vi "test_request_builder_api.vi"() -> ()   [LabVIEW 2020, in "reqwest_tests.lvlib"]
uses:
  reqwest_tests.lvlib
  <vilib>/addons/_JKI Toolkits/Caraya/classes/Assert/Assert.lvclass
  <vilib>/addons/_JKI Toolkits/Caraya/classes/Test/Test.lvclass
  ClientBuilder/ClientBuilder.lvclass
  Client/Client.lvclass
  Types/http_method_enum.ctl
  reqwest.lvlib
  RequestBuilder/RequestBuilder.lvclass
  Headers/Headers.lvclass
  Request/Request.lvclass
panel:
  out "string_value":string
  out "is_complete":bool
  in  "error in (no error)":errorcluster
  out "error out":errorcluster
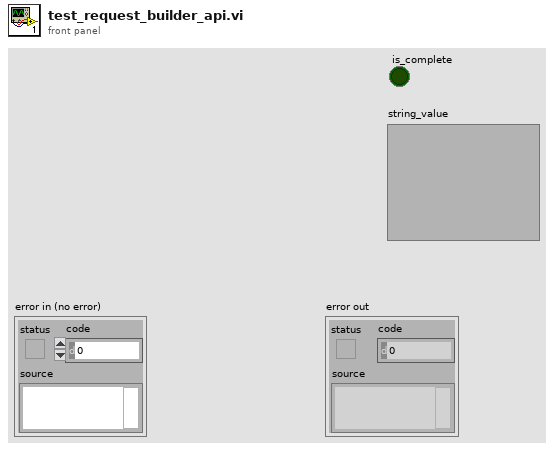
[diagram p1: front panel]
types:
  T1 = typedef "reqwest.lvlib/http_method_enum.ctl" = enum8{"<select>", "GET", "POST", "PUT", "DELETE", "HEAD", "OPTIONS", "CONNECT", "PATCH", "TRACE"}
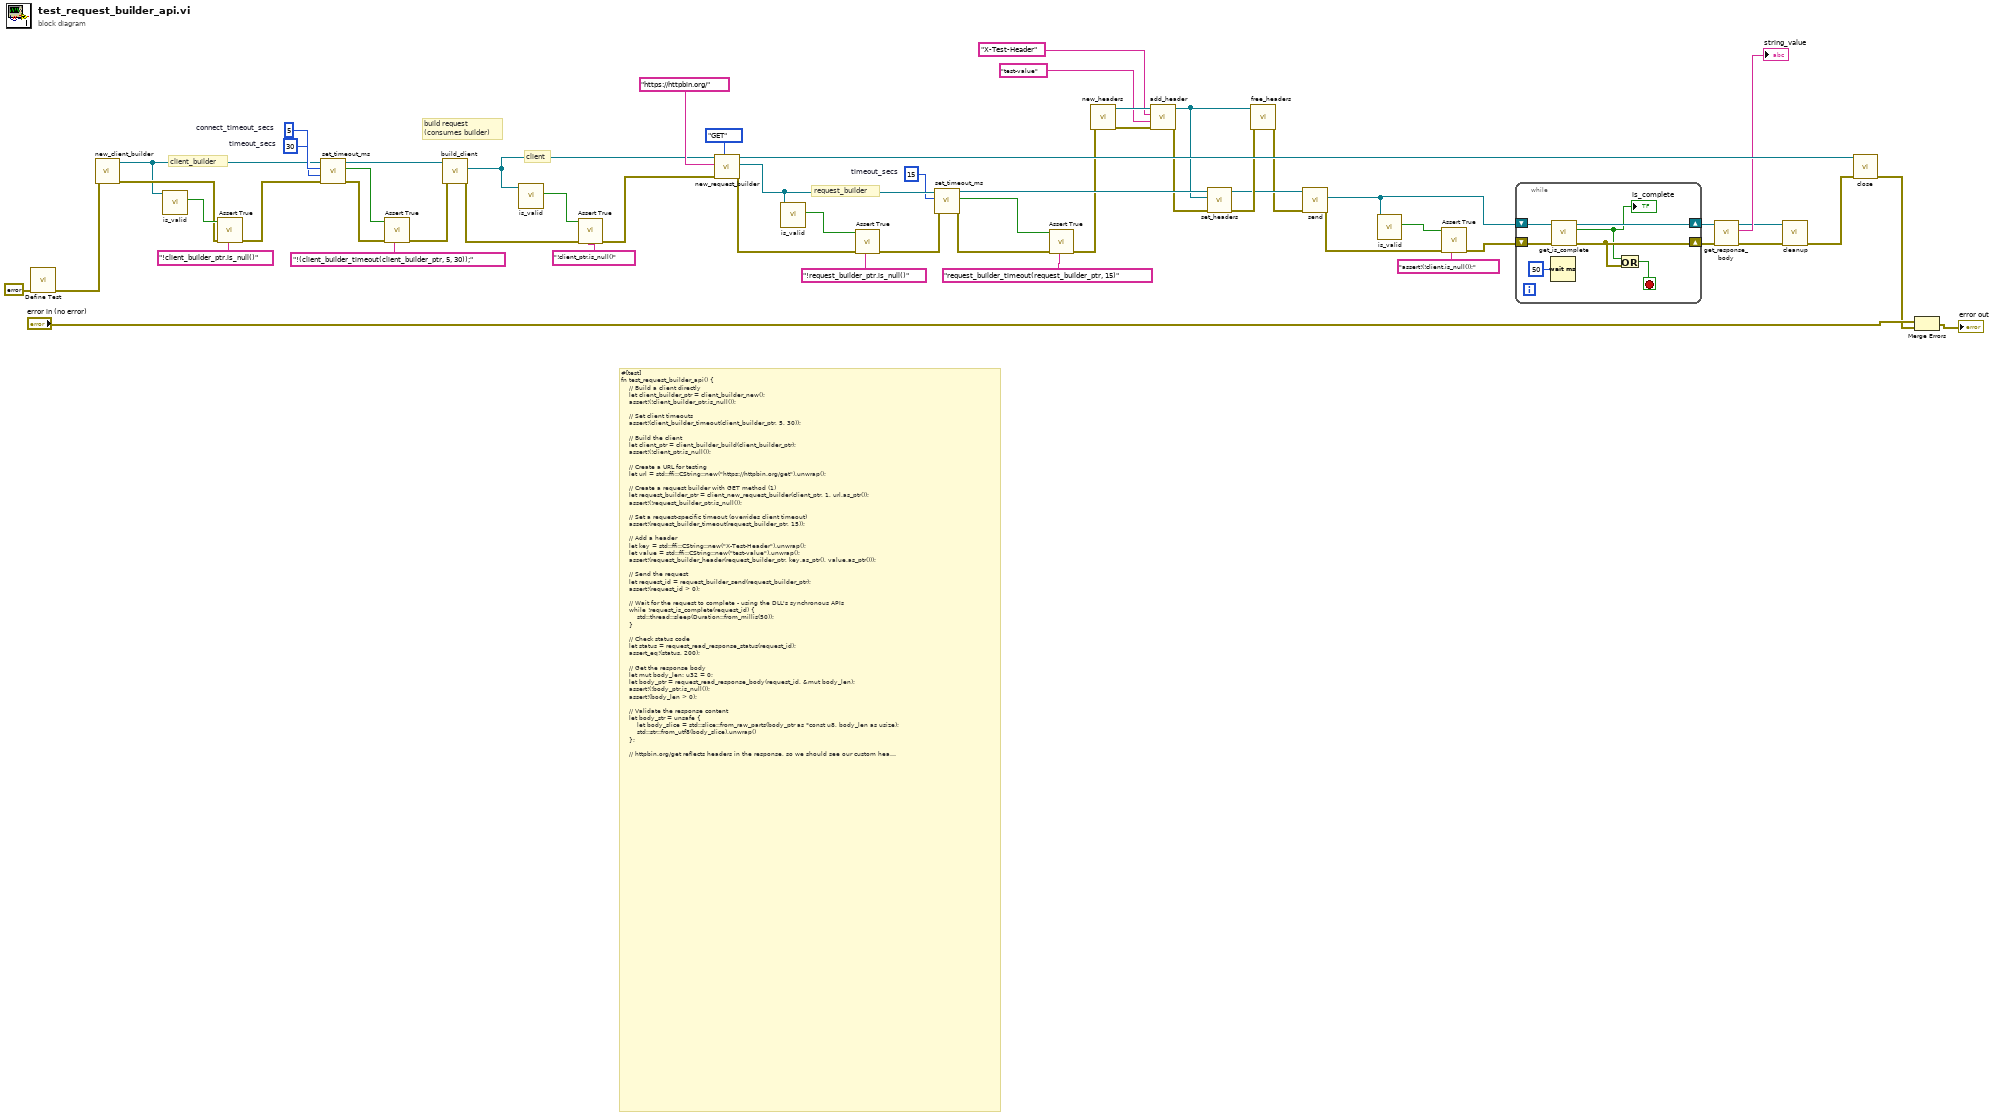
[diagram p0: block diagram]
diagram:
  w30 = u64 15  # timeout_secs
  w45 = u64 30  # timeout_secs
  w46 = u64 5  # connect_timeout_secs
  # "request_builder"
  # "client"
  # "client_builder"
  # "build request\n(consumes builder)"
  # "#[test]\nfn test_request_builder_api() {\n    // Build a client directly \n    let client_builder_ptr = client_builder_new();\n    assert!(!client_builder_ptr.is_null());\n    \n    // Set client timeouts\n    assert!(client_builder_timeout(client_builder_ptr, 5, 30));\n    \n    // Build the client\n    let client_ptr = client_builder_build(client_builder_ptr);\n    assert!(!client_ptr.is_null());\n\n    // Create a URL for testing\n    let url = std::ffi::CString::new(\"https://httpbin.org/get\").unwrap();\n    \n    // Create a request builder with GET method (1)\n    let request_builder_ptr = client_new_request_builder(client_ptr, 1, url.as_ptr());\n    assert!(!request_builder_ptr.is_null());\n    \n    // Set a request-specific timeout (overrides client timeout)\n    assert!(request_builder_timeout(request_builder_ptr, 15));\n    \n    // Add a header\n    let key = std::ffi::CString::new(\"X-Test-Header\").unwrap();\n    let value = std::ffi::CString::new(\"test-value\").unwrap();\n    assert!(request_builder_header(request_builder_ptr, key.as_ptr(), value.as_ptr()));\n    \n    // Send the request\n    let request_id = request_builder_send(request_builder_ptr);\n    assert!(request_id > 0);\n    \n    // Wait for the request to complete - using the DLL's synchronous APIs\n    while !request_is_complete(request_id) {\n        std::thread::sleep(Duration::from_millis(50));\n    }\n    \n    // Check status code\n    let status = request_read_response_status(request_id);\n    assert_eq!(status, 200);\n    \n    // Get the response body\n    let mut body_len: u32 = 0;\n    let body_ptr = request_read_response_body(request_id, &mut body_len);\n    assert!(!body_ptr.is_null());\n    assert!(body_len > 0);\n    \n    // Validate the response content\n    let body_str = unsafe {\n        let body_slice = std::slice::from_raw_parts(body_ptr as *const u8, body_len as usize);\n        std::str::from_utf8(body_slice).unwrap()\n    };\n    \n    // httpbin.org/get reflects headers in the response, so we should see our custom header\n    assert!(body_str.contains(\"X-Test-Header\"));\n    assert!(body_str.contains(\"test-value\"));\n    \n    // Cleanup\n    free_memory(body_ptr);\n    request_cleanup(request_id);\n    client_close(client_ptr);\n}"
  n1 = call <vilib>:"Define Test.vi"("error in (no error)"=errorcluster {"status"=FALSE, "code"=0, "source"=""}) -> ("error out"=w48:errorcluster)  [unwired: 9 in, 1 out]
  n2 = call "new_client_builder.vi"("error in (no error)"=w48) -> ("error out"=w47:errorcluster, "Client out"=w41:refnum<class "ClientBuilder.lvclass">)  [unwired: 9 in]
  n3 = call "is_valid.vi"("Client in"=w41) -> ("valid-ref?"=w53:bool)  [unwired: 10 in]
  n4 = call <vilib>:"Assert True.vi"("Label"="!client_builder_ptr.is_null()", "error in (no error)"=w47, "True?"=w53) -> ("error out"=w40:errorcluster)  [unwired: 7 in, 1 out]
  n5 = call "set_timeout_ms.vi"("error in (no error)"=w40, "timeout_secs"=w45, 10:w46, "ClientBuilder in"=w41) -> ("error out"=w42:errorcluster, "success"=w43:bool, "ClientBuilder out"=w38:refnum<class "ClientBuilder.lvclass">)  [unwired: 5 in]
  n6 = call <vilib>:"Assert True.vi"("Label"="!(client_builder_timeout(client_builder_ptr, 5, 30));", "error in (no error)"=w42, "True?"=w43) -> ("error out"=w26:errorcluster)  [unwired: 7 in, 1 out]
  n7 = call "build_client.vi"("error in (no error)"=w26, "ClientBuilder in"=w38) -> ("error out"=w25:errorcluster, "Client out"=w34:refnum<class "Client.lvclass">)  [unwired: 8 in]
  n8 = call "is_valid.vi"("Client in"=w34) -> ("valid-ref?"=w51:bool)  [unwired: 10 in]
  n9 = call <vilib>:"Assert True.vi"("Label"="!client_ptr.is_null()", "error in (no error)"=w25, "True?"=w51) -> ("error out"=w32:errorcluster)  [unwired: 7 in, 1 out]
  n10 = call "new_request_builder.vi"("HTTP Method"=http_method_enum."GET", "error in (no error)"=w32, "url"="https://httpbin.org/" ("Label"), "Client in"=w34) -> ("error out"=w24:errorcluster, "RequestBuilder out"=w31:refnum<class "RequestBuilder.lvclass">, "Client out"=w33:refnum<class "Client.lvclass">)  [unwired: 5 in]
  n11 = call "is_valid.vi"("obj in"=w31) -> ("valid-ref?"=w35:bool)  [unwired: 10 in]
  n12 = call <vilib>:"Assert True.vi"("Label"="!request_builder_ptr.is_null()", "error in (no error)"=w24, "True?"=w35) -> ("error out"=w23:errorcluster)  [unwired: 7 in, 1 out]
  n13 = call "set_timeout_ms.vi"("error in (no error)"=w23, "timeout_ms"=w30, "obj in"=w31) -> ("error out"=w27:errorcluster, "success"=w28:bool, "obj out"=w22:refnum<class "RequestBuilder.lvclass">)  [unwired: 6 in]
  n14 = call <vilib>:"Assert True.vi"("Label"="request_builder_timeout(request_builder_ptr, 15)", "error in (no error)"=w27, "True?"=w28) -> ("error out"=w15:errorcluster)  [unwired: 7 in, 1 out]
  n15 = call "new_headers.vi"("error in (no error)"=w15) -> ("error out"=w18:errorcluster, "Headers out"=w21:refnum<class "Headers.lvclass">)  [unwired: 9 in]
  n16 = call "add_header.vi"("error in (no error)"=w18, "value"="test-value" ("Label"), "key"="X-Test-Header" ("Label"), "Headers in"=w21) -> ("error out"=w16:errorcluster, "Headers out"=w17:refnum<class "Headers.lvclass">)  [unwired: 5 in, 1 out]
  n17 = call "set_headers.vi"("error in (no error)"=w16, "Headers"=w17, "obj in"=w22) -> ("error out"=w14:errorcluster, "obj out"=w13:refnum<class "RequestBuilder.lvclass">)  [unwired: 6 in, 1 out]
  n18 = call "free_headers.vi"("error in (no error)"=w14, "Headers in"=w17) -> ("error out"=w5:errorcluster)  [unwired: 9 in]
  n19 = call "send.vi"("error in (no error)"=w5, "obj in"=w13) -> ("error out"=w4:errorcluster, "request"=w6:refnum<class "Request.lvclass">)  [unwired: 8 in]
  n20 = call "is_valid.vi"("Request in"=w6) -> ("valid-ref?"=w11:bool)  [unwired: 10 in]
  n21 = call <vilib>:"Assert True.vi"("Label"="assert!(!client.is_null());", "error in (no error)"=w4, "True?"=w11) -> ("error out"=w10:errorcluster)  [unwired: 7 in, 1 out]
  n22 = while {
    shift-right: [w63] -> w7
    shift-left: w6 -> [w62]
    shift-right: [w59] -> w9
    shift-left: w10 -> [w60]
    stop <- w57 stop-if-true
    n23 = Wait (ms)(milliseconds to wait=u32 50) -> ()  [unwired: 1 out]
    n24 = call "get_is_complete.vi"("error in (no error)"=w60, "Request in"=w62) -> ("error out"=w59:errorcluster, "is_complete"=w58:bool, "Request out"=w63:refnum<class "Request.lvclass">)  [unwired: 7 in]
    "is_complete" <- w58
    n25 = Or(x=w58, y=w59) -> (x .or. y?=w57:bool)
  }
  n26 = call "get_response_body.vi"("error in (no error)"=w9, "Request in"=w7) -> ("error out"=w2:errorcluster, "string_value"=→"string_value":string, "Request in"=w3:refnum<class "Request.lvclass">)  [unwired: 7 in]
  n27 = call "cleanup.vi"("error in (no error)"=w2, "Request in"=w3) -> ("error out"=w1:errorcluster)  [unwired: 8 in, 1 out]
  n28 = call "close.vi"("error in (no error)"=w1, "Client in"=w33) -> ("error out"=w49:errorcluster)  [unwired: 9 in]
  n29 = Merge Errors("error in (no error)", w49) -> (→"error out":errorcluster)
